vi "Flatten.vi"(8 "error in (no error)":errorcluster, 11 "ClusterMessagePacket in":refnum<class "ClusterMessagePacket.lvclass">) -> (0 "error out":errorcluster, 3 "Flattened Packet":string)   [LabVIEW 2020, in "Network Messenger.lvlib" / "ClusterMessagePacket.lvclass"]
uses:
  <vilib>/gpm_packages/@cs/Network-interface/Source/Network Messenger/ClusterMessagePacket/ClusterMessagePacket.lvclass
  <vilib>/gpm_packages/@cs/Network-interface/Source/Network Messenger/ClusterMessagePacket/ClusterMessagePacket.lvclass/ClusterMessagePacket.ctl
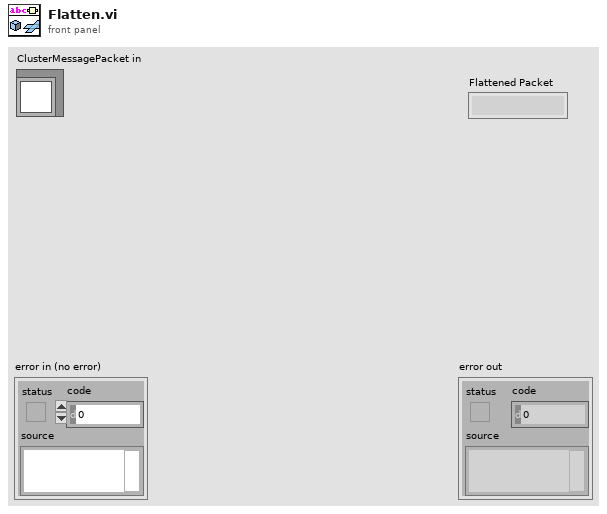
[diagram p1: front panel]
types:
  T1 = typedef "Network Messenger.lvlib/Message Packet.ctl" = cluster{"Msg":string, "Data":variant}
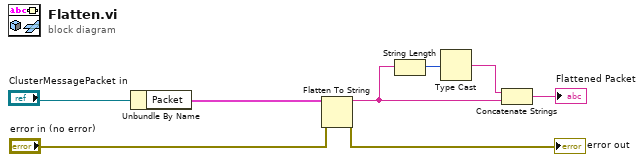
[diagram p0: block diagram]
diagram:
  n1 = Unbundle By Name("ClusterMessagePacket in") -> ("Packet"=w1:T1)
  n2 = Flatten To String(anything=w1, error in (no error)="error in (no error)") -> (data string=w5:string, error out=→"error out":errorcluster)  [unwired: 2 in, 1 out]
  n3 = String Length(string=w5) -> (length=w4:i32)
  n4 = Type Cast(x=w4) -> (*(type *) &x=w2:string)  [unwired: 1 in]
  n5 = Concatenate Strings(w2, w5) -> (→"Flattened Packet":string)
